vi "XY_sequence_generator2.vi"(8 "X-direction":enum16{"Up", "Down"}(ring), 9 "Y-direction":enum16{"Left", "Right"}(ring)=enum."Right", 10 "Acquisition time (ms)":dbl, 11 "XY acquisition":T1={"Number of tiles in X"=3.0, "Number of tiles in Y"=3.0, "Step size XY (µm)"=500.0, "Acquire XY-tiling"=FALSE, "Moving time (ms)"=1000.0}) -> (3 "string array":string[](array[string]))   [LabVIEW 2020]
uses:
  typedefs/typedef_XY_tiling.ctl
panel:
  out "String":string
  in  "fast axis":enum16{"", "X-axis", "Y-axis"}(ring)
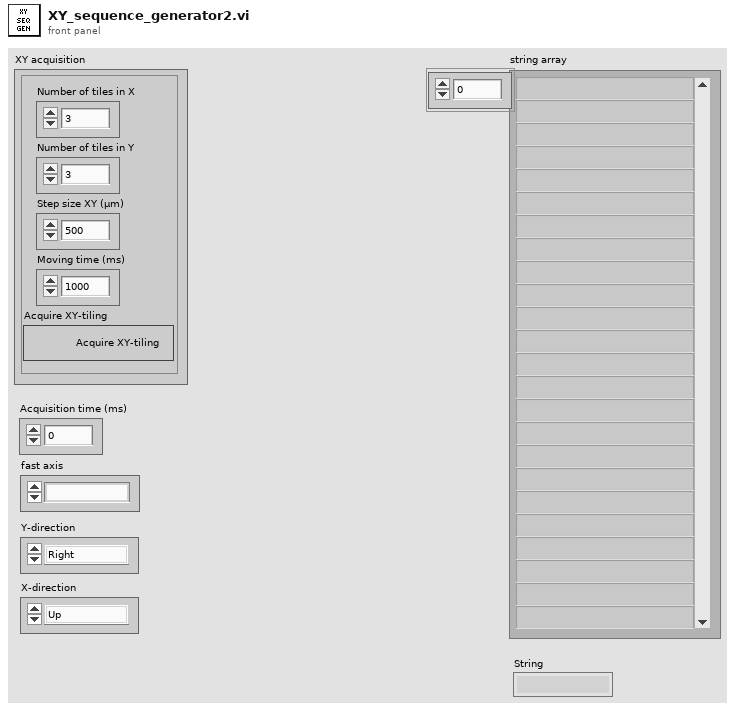
[diagram p1: front panel]
types:
  T1 = typedef "typedef_XY_tiling.ctl" = cluster{"Number of tiles in X":dbl, "Number of tiles in Y":dbl, "Step size XY (µm)":dbl, "Acquire XY-tiling":bool, "Moving time (ms)":dbl}
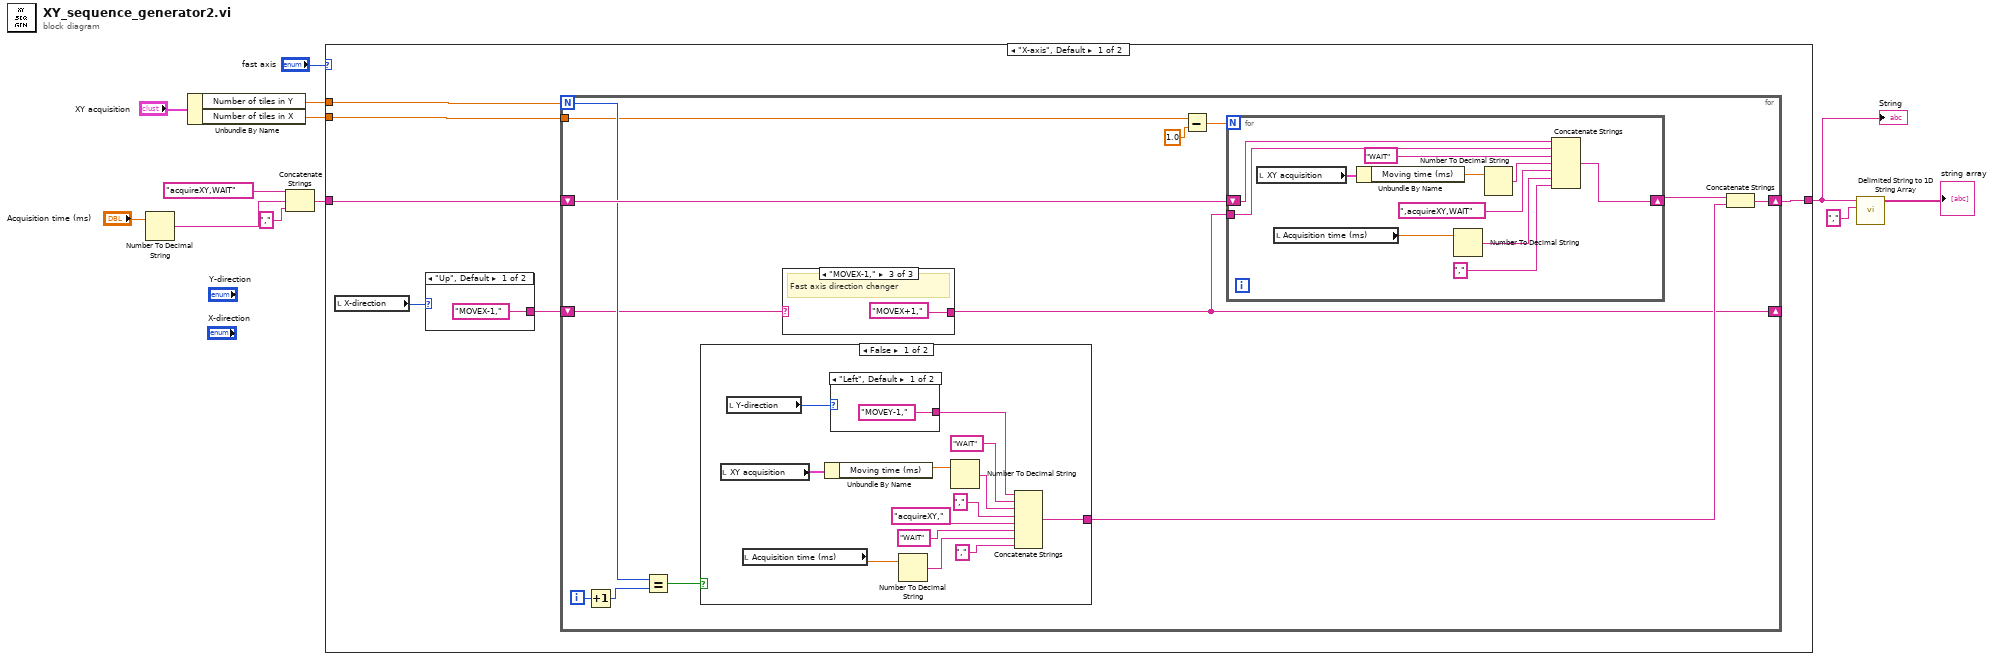
[diagram p0: block diagram]
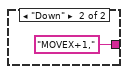
[diagram p2: hidden frame]
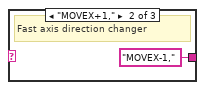
[diagram p4: hidden frame]
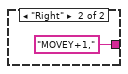
[diagram p5: hidden frame]
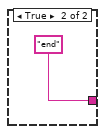
[diagram p6: hidden frame]
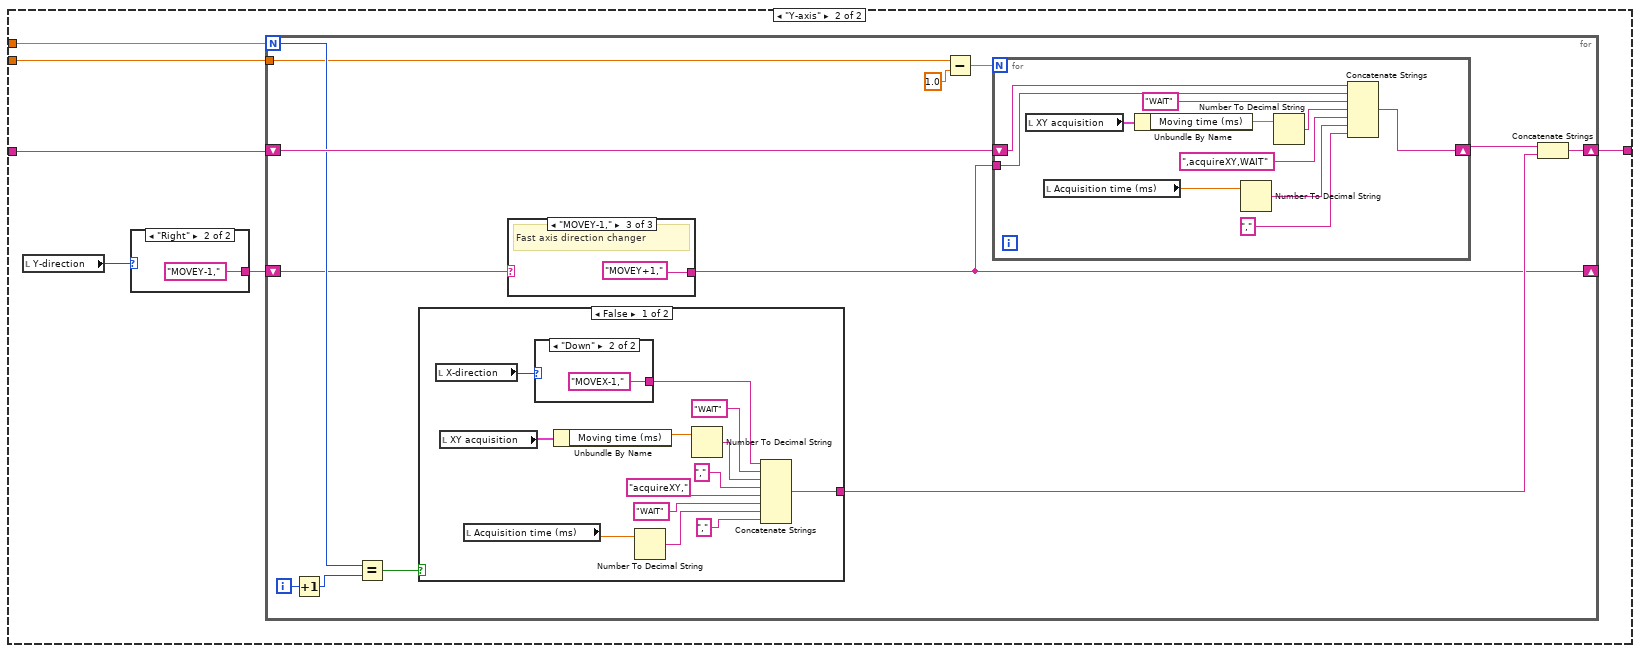
[diagram p7: hidden frame]
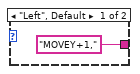
[diagram p8: hidden frame]
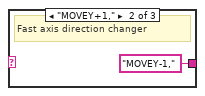
[diagram p10: hidden frame]
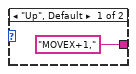
[diagram p11: hidden frame]
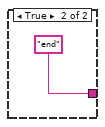
[diagram p12: hidden frame]
diagram:
  n1 = Number To Decimal String(number="Acquisition time (ms)") -> (decimal integer string=w4:string)  [unwired: 1 in]
  n2 = Unbundle By Name("XY acquisition") -> ("Number of tiles in Y"=w7:dbl, "Number of tiles in X"=w8:dbl)
  n3 = Concatenate Strings("acquireXY,WAIT", w4, "," ("string")) -> (w2:string)
  n4 = case shown="\"X-axis\", Default" "fast axis" {
    tunnel: [w18 w68] -> w11
    tunnel: w8 -> [w17 w67]
    tunnel: w7 -> [w16 w66]
    tunnel: w2 -> [w15 w65]
    frame "X-axis", Default {
      n5 = local read "X-direction"() -> (w14:enum16{"Up", "Down"})
      n6 = case shown="\"Up\", Default" w14 {
        tunnel: ["MOVEX-1," "MOVEX+1,"] -> w13
        frame "Up", Default {
        }
        frame "Down" {
        }
      }
      n7 = for {
        N: w16 -> [w29]
        tunnel: w17 -> [w22]
        shift-right: [w31] -> w18
        shift-left: w15 -> [w33]
        shift-right: [w24] -> _
        shift-left: w13 -> [w25]
        i -> [w26]
        n8 = Increment(x=w26) -> (x+1=w27:i32)
        n9 = Equal?(x=w29, y=w27) -> (x = y?=w30:bool)
        n10 = case shown="False" w30 {
          tunnel: [w44 "end" ("string")] -> w28
          frame False {
            n11 = local read "XY acquisition"() -> (w45:T1)
            n12 = local read "Y-direction"() -> (w37:enum16{"Left", "Right"})
            n13 = local read "Acquisition time (ms)"() -> (w42:dbl)
            n14 = Unbundle By Name(w45) -> ("Moving time (ms)"=w47:dbl)
            n15 = case shown="\"Left\", Default" w37 {
              tunnel: ["MOVEY-1," "MOVEY+1,"] -> w36
              frame "Left", Default {
              }
              frame "Right" {
              }
            }
            n16 = Number To Decimal String(number=w42) -> (decimal integer string=w39:string)  [unwired: 1 in]
            n17 = Number To Decimal String(number=w47) -> (decimal integer string=w46:string)  [unwired: 1 in]
            n18 = Concatenate Strings(w36, "WAIT" ("string"), w46, "," ("string"), "acquireXY," ("string"), "WAIT" ("string"), w39, "," ("string")) -> (w44:string)
          }
          frame True {
          }
        }
        n19 = case shown="\"MOVEX-1,\"" w25 {
          tunnel: [_ "MOVEX-1," "MOVEX+1,"] -> w24
          frame "False", Default {
          }
          frame "MOVEX+1," {
            # "Fast axis direction changer"
          }
          frame "MOVEX-1," {
            # "Fast axis direction changer"
          }
        }
        n20 = Subtract(x=w22, y=1.0) -> (x-y=w23:dbl)
        n21 = for {
          N: w23 -> [_]
          shift-right: [w62] -> w32
          shift-left: w33 -> [w59]
          tunnel: w24 -> [w58]
          n22 = local read "XY acquisition"() -> (w61:T1)
          n23 = local read "Acquisition time (ms)"() -> (w54:dbl)
          n24 = Unbundle By Name(w61) -> ("Moving time (ms)"=w60:dbl)
          n25 = Number To Decimal String(number=w54) -> (decimal integer string=w53:string)  [unwired: 1 in]
          n26 = Number To Decimal String(number=w60) -> (decimal integer string=w56:string)  [unwired: 1 in]
          n27 = Concatenate Strings(w59, w58, "WAIT" ("string"), w56, ",acquireXY,WAIT" ("string"), w53, "," ("string")) -> (w62:string)
        }
        n28 = Concatenate Strings(w32, w28) -> (w31:string)
      }
    }
    frame "Y-axis" {
      n29 = local read "Y-direction"() -> (w64:enum16{"Left", "Right"})
      n30 = case shown="\"Right\"" w64 {
        tunnel: ["MOVEY+1," "MOVEY-1,"] -> w63
        frame "Left", Default {
        }
        frame "Right" {
        }
      }
      n31 = for {
        N: w66 -> [w79]
        tunnel: w67 -> [w72]
        shift-right: [w81] -> w68
        shift-left: w65 -> [w83]
        shift-right: [w74] -> _
        shift-left: w63 -> [w75]
        i -> [w76]
        n32 = Increment(x=w76) -> (x+1=w77:i32)
        n33 = Equal?(x=w79, y=w77) -> (x = y?=w80:bool)
        n34 = case shown="False" w80 {
          tunnel: [w94 "end" ("string")] -> w78
          frame False {
            n35 = local read "X-direction"() -> (w87:enum16{"Up", "Down"})
            n36 = local read "XY acquisition"() -> (w95:T1)
            n37 = local read "Acquisition time (ms)"() -> (w92:dbl)
            n38 = case shown="\"Down\"" w87 {
              tunnel: ["MOVEX+1," "MOVEX-1,"] -> w86
              frame "Up", Default {
              }
              frame "Down" {
              }
            }
            n39 = Unbundle By Name(w95) -> ("Moving time (ms)"=w97:dbl)
            n40 = Number To Decimal String(number=w92) -> (decimal integer string=w89:string)  [unwired: 1 in]
            n41 = Number To Decimal String(number=w97) -> (decimal integer string=w96:string)  [unwired: 1 in]
            n42 = Concatenate Strings(w86, "WAIT" ("string"), w96, "," ("string"), "acquireXY," ("string"), "WAIT" ("string"), w89, "," ("string")) -> (w94:string)
          }
          frame True {
          }
        }
        n43 = case shown="\"MOVEY-1,\"" w75 {
          tunnel: [_ "MOVEY-1," "MOVEY+1,"] -> w74
          frame "False", Default {
          }
          frame "MOVEY+1," {
            # "Fast axis direction changer"
          }
          frame "MOVEY-1," {
            # "Fast axis direction changer"
          }
        }
        n44 = Subtract(x=w72, y=1.0) -> (x-y=w73:dbl)
        n45 = for {
          N: w73 -> [_]
          shift-right: [w112] -> w82
          shift-left: w83 -> [w109]
          tunnel: w74 -> [w108]
          n46 = local read "XY acquisition"() -> (w111:T1)
          n47 = local read "Acquisition time (ms)"() -> (w104:dbl)
          n48 = Unbundle By Name(w111) -> ("Moving time (ms)"=w110:dbl)
          n49 = Number To Decimal String(number=w104) -> (decimal integer string=w103:string)  [unwired: 1 in]
          n50 = Number To Decimal String(number=w110) -> (decimal integer string=w106:string)  [unwired: 1 in]
          n51 = Concatenate Strings(w109, w108, "WAIT" ("string"), w106, ",acquireXY,WAIT" ("string"), w103, "," ("string")) -> (w112:string)
        }
        n52 = Concatenate Strings(w82, w78) -> (w81:string)
      }
    }
  }
  "String" <- w11
  n53 = call <vilib>:"Delimited String to 1D String Array.vi"("delimiter"=",", "delimited string"=w11) -> ("string array"=→"string array":string[])  [unwired: 9 in]
